vi "Script Cases.vi"(0 "primitive":i32, 1 "argument 1":dbl, 2 "argument 2":dbl, 3 "argument 3":dbl, 4 "argument 4":dbl, 5 "argument 5":dbl) -> ()   [LabVIEW 2014]
uses:
  Begin/Global Variables.vi
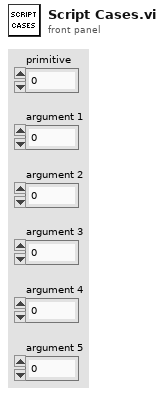
[diagram p1: front panel]
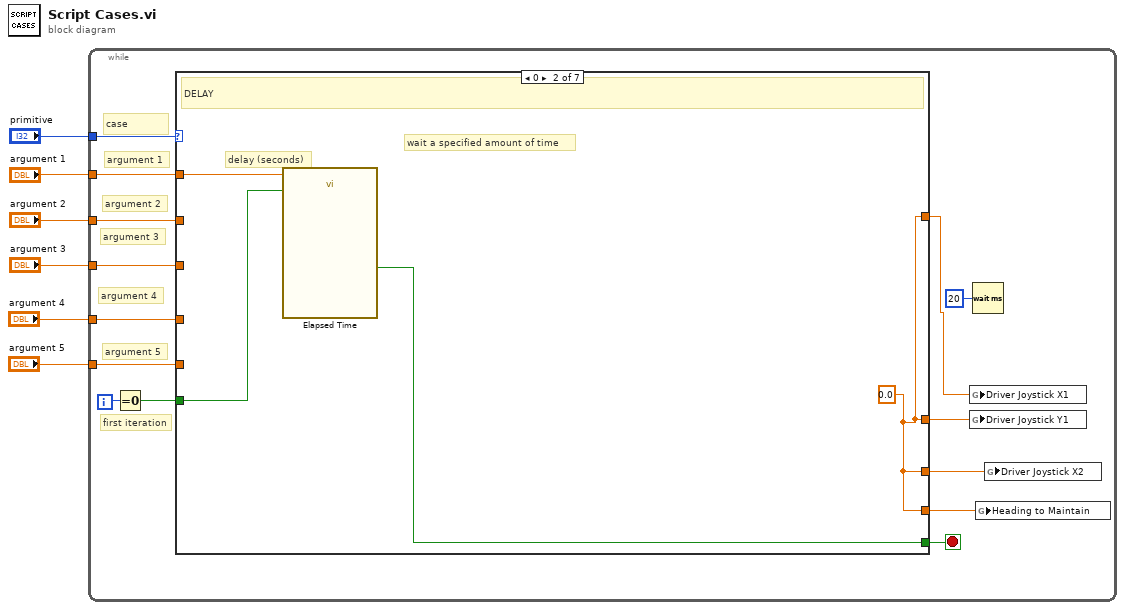
[diagram p0: block diagram]
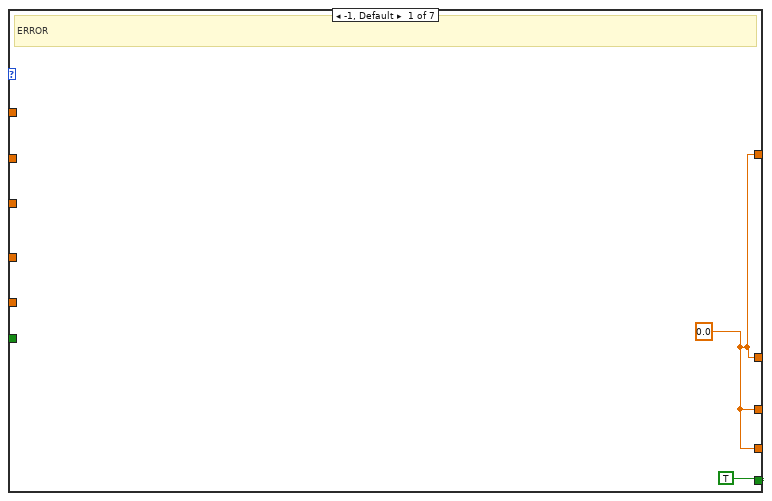
[diagram p2: hidden frame]
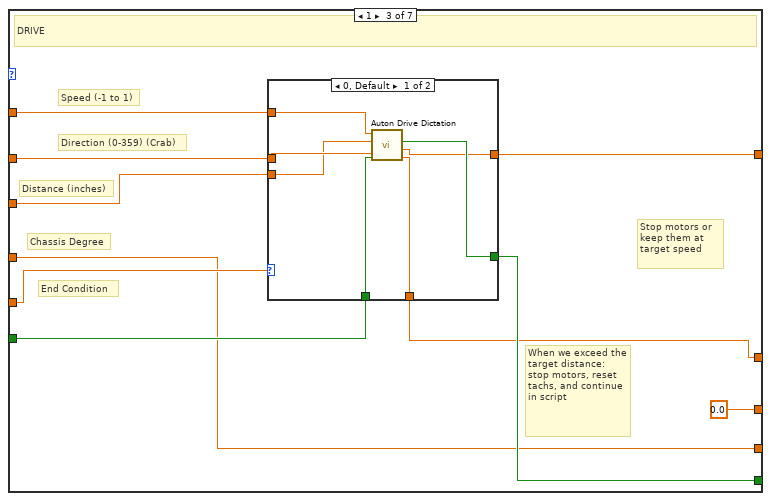
[diagram p3: hidden frame]
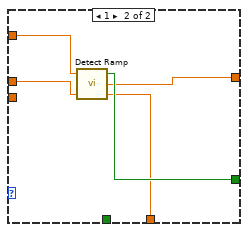
[diagram p4: hidden frame]
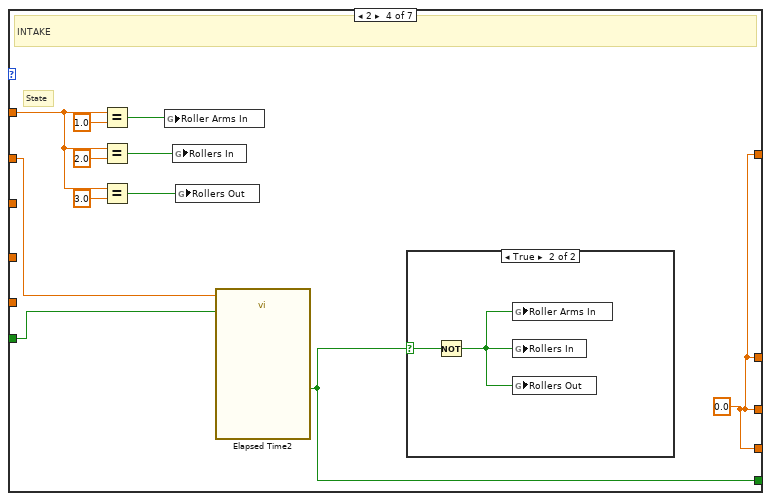
[diagram p5: hidden frame]
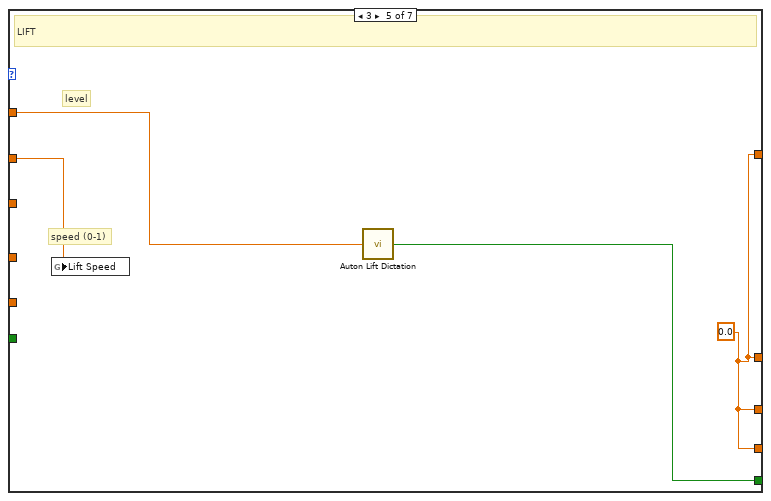
[diagram p7: hidden frame]
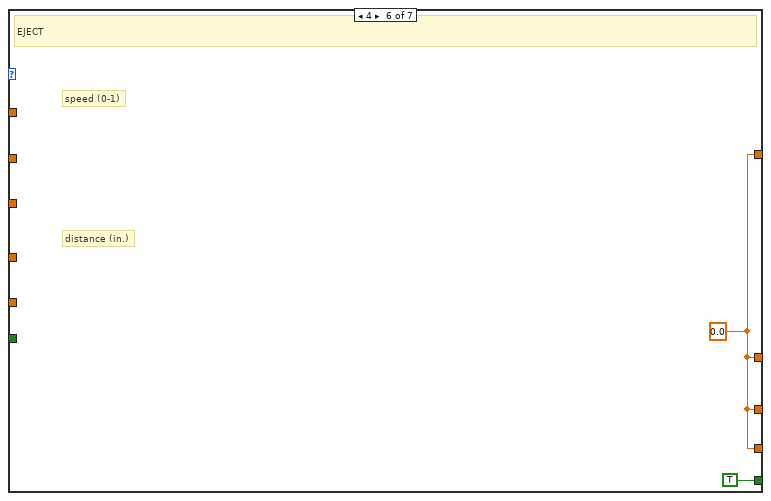
[diagram p8: hidden frame]
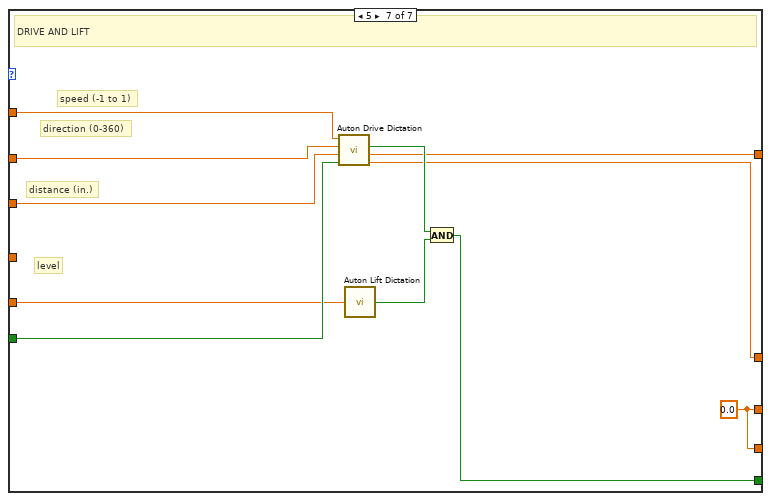
[diagram p9: hidden frame]
diagram:
  n1 = while {
    tunnel: "argument 1" -> [w20]
    tunnel: "argument 2" -> [w19]
    tunnel: "argument 3" -> [w18]
    tunnel: "argument 4" -> [w17]
    tunnel: "argument 5" -> [w16]
    tunnel: "primitive" -> [w15]
    i -> [w13]
    stop <- w14 stop-if-true
    # "first iteration"
    # "case"
    # "argument 5"
    # "argument 4"
    # "argument 3"
    # "argument 2"
    # "argument 1"
    n2 = Equal To 0?(x=w13) -> (x = 0?=w12:bool)
    n3 = case shown="0" w15 {
      tunnel: w20 -> [_ w26 w35 w56 w64 _ w77]
      tunnel: w19 -> [_ _ w34 w52 w65 _ w76]
      tunnel: w18 -> [_ _ w33 _ _ _ w75]
      tunnel: w17 -> [_ _ w29 _ _ _ _]
      tunnel: w16 -> [_ _ w30 _ _ _ w73]
      tunnel: [TRUE w24 w32 w51 w63 TRUE w70] -> w14
      tunnel: w12 -> [_ w25 w31 w50 _ _ w74]
      tunnel: [w21 w23 0.0 ("argument 1") w49 w62 w66 w78] -> w11
      tunnel: [w21 w23 w29 w49 w62 w66 w78] -> w10
      tunnel: [w21 w23 w28 w49 w62 w66 w69] -> w8
      tunnel: [w21 w23 w27 w49 w62 w66 w68] -> w7
      frame -1, Default {
        w21 = 0.0 ("argument 1")
        # "ERROR"
      }
      frame 0 {
        w23 = 0.0 ("argument 1")
        # "wait a specified amount of time"
        # "delay (seconds)"
        # "DELAY"
        n4 = call "Elapsed Time"("Time Target (s)"=w26, "Reset"=w25) -> ("Time has Elapsed"=w24:bool)  [unwired: 10 in, 7 out]
      }
      frame 1 {
        # "Chassis Degree"
        # "End Condition"
        # "When we exceed the target distance: stop motors, reset tachs, and continue in script"
        # "Stop motors or keep them at target speed"
        # "Distance (inches)"
        # "Direction (0-359) (Crab)"
        # "Speed (-1 to 1)"
        # "DRIVE"
        n5 = case shown="0, Default" w30 {
          tunnel: w35 -> [w43 w48]
          tunnel: w34 -> [w42 w47]
          tunnel: w33 -> [w41 _]
          tunnel: [w40 w46] -> w32
          tunnel: w31 -> [w39 _]
          tunnel: [w38 w45] -> w28
          tunnel: [w37 w44] -> w27
          frame 0, Default {
            n6 = call "Auton Drive Dictation.vi"("Reset Encoders"=w39, "Distance (inches)"=w41, "Direction (0-359)"=w42, "Speed (0 to 1)"=w43) -> ("Joy Y"=w37:dbl, "Joy X"=w38:dbl, "Distance Reached?"=w40:bool)  [unwired: 5 in]
          }
          frame 1 {
            n7 = call "Detect Ramp.vi"("Direction"=w47, "Speed"=w48) -> ("JoyY"=w44:dbl, "Joy X"=w45:dbl, "Finished"=w46:bool)  [unwired: 1 in]
          }
        }
      }
      frame 2 {
        w49 = 0.0 ("argument 1")
        # "State"
        # "INTAKE"
        n8 = Equal?(x=w56, y=1.0) -> (x = y?=w53:bool)
        n9 = Equal?(x=w56, y=2.0) -> (x = y?=w54:bool)
        n10 = Equal?(x=w56, y=3.0) -> (x = y?=w55:bool)
        n11 = global write "Global Variables.vi" "Roller Arms In"(w53) -> ()
        n12 = global write "Global Variables.vi" "Rollers In"(w54) -> ()
        n13 = global write "Global Variables.vi" "Rollers Out"(w55) -> ()
        n14 = call "Elapsed Time2"("Time Target (s)"=w52, "Reset"=w50) -> ("Time has Elapsed"=w51:bool)  [unwired: 10 in, 7 out]
        n15 = case shown="True" w51 {
          selector: w51 -> [_ w61]
          frame False {
          }
          frame True {
            n16 = Not(x=w61) -> (.not. x?=w60:bool)
            n17 = global write "Global Variables.vi" "Roller Arms In"(w60) -> ()
            n18 = global write "Global Variables.vi" "Rollers In"(w60) -> ()
            n19 = global write "Global Variables.vi" "Rollers Out"(w60) -> ()
          }
        }
      }
      frame 3 {
        w62 = 0.0 ("argument 1")
        # "speed (0-1)"
        # "level"
        # "LIFT"
        n20 = global write "Global Variables.vi" "Lift Speed"(w65) -> ()
        n21 = call "Auton Lift Dictation.vi"("Level"=w64) -> ("Lift Sequence Done"=w63:bool)
      }
      frame 4 {
        w66 = 0.0 ("argument 1")
        # "distance (in.)"
        # "speed (0-1)"
        # "EJECT"
      }
      frame 5 {
        w78 = 0.0 ("argument 1")
        # "level"
        # "distance (in.)"
        # "direction (0-360)"
        # "speed (-1 to 1)"
        # "DRIVE AND LIFT"
        n22 = call "Auton Drive Dictation.vi"("Reset Encoders"=w74, "Distance (inches)"=w75, "Direction (0-359)"=w76, "Speed (0 to 1)"=w77) -> ("Joy Y"=w68:dbl, "Joy X"=w69:dbl, "Distance Reached?"=w72:bool)  [unwired: 5 in]
        n23 = call "Auton Lift Dictation.vi"("Level"=w73) -> ("Lift Sequence Done"=w71:bool)
        n24 = And(x=w72, y=w71) -> (x .and. y?=w70:bool)
      }
    }
    n25 = global write "Global Variables.vi" "Driver Joystick X1"(w8) -> ()
    n26 = global write "Global Variables.vi" "Driver Joystick Y1"(w7) -> ()
    n27 = Wait (ms)(milliseconds to wait=u32 20) -> ()  [unwired: 1 out]
    n28 = global write "Global Variables.vi" "Heading to Maintain"(w10) -> ()
    n29 = global write "Global Variables.vi" "Driver Joystick X2"(w11) -> ()
  }
